vi "1_PrendeLed_Boton.vi"() -> ()   [LabVIEW 2020]
panel:
  out "Boolean array":bool[](array[boolean])
  in  "stop":bool
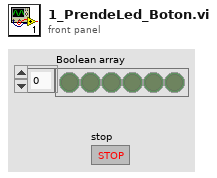
[diagram p1: front panel]
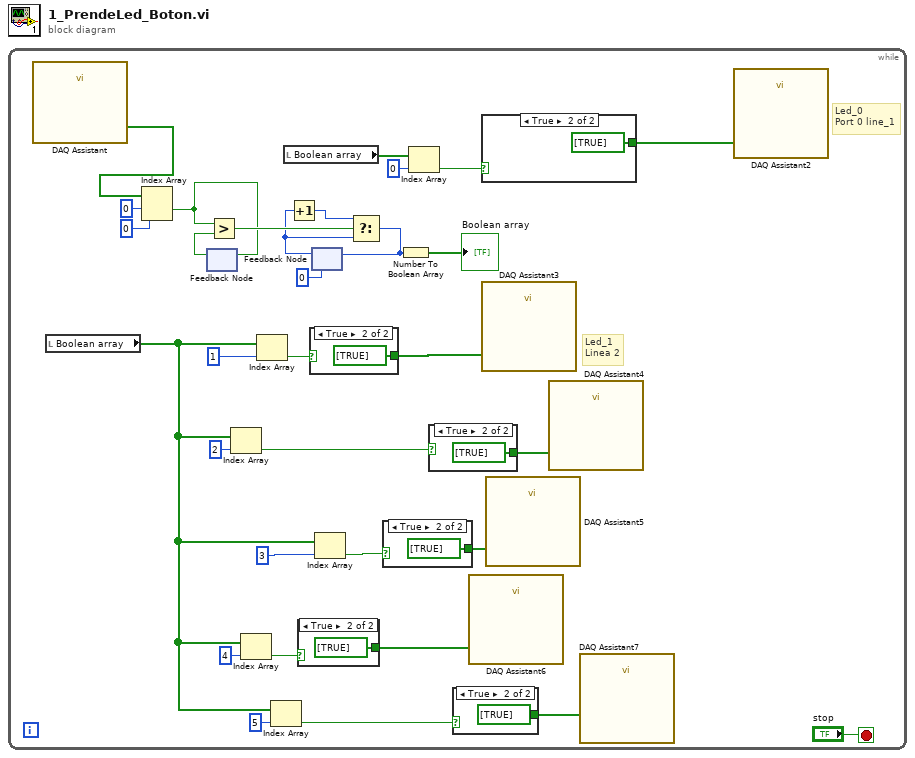
[diagram p0: block diagram]
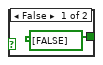
[diagram p2: hidden frame]
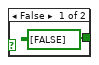
[diagram p3: hidden frame]
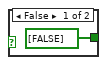
[diagram p4: hidden frame]
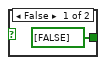
[diagram p5: hidden frame]
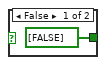
[diagram p6: hidden frame]
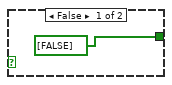
[diagram p7: hidden frame]
diagram:
  n1 = while {
    stop <- "stop" stop-if-true
    # "Led_0\nPort 0 line_1"
    # "Led_1\nLinea 2"
    n2 = call "DAQ Assistant"() -> ("data"=w7:bool[])  [unwired: 17 in, 2 out]
    n3 = local read "Boolean array"() -> (w15:bool[])
    n4 = Index Array(array=w7, index #1=0 ("index"), index #2=0 ("index")) -> (element #1=w9:bool)  [unwired: 1 out]
    n5 = feedback #1() -> (w13:bool)  [unwired: 1 in]
    n6 = feedback-in #1(w9) -> ()
    n7 = Greater?(x=w9, y=w13) -> (0:w14:bool)
    n8 = Index Array(array=w15, index=2) -> (element=w22:bool)
    n9 = Index Array(array=w15, index=4) -> (element=w18:bool)
    n10 = Index Array(array=w15, index=1) -> (element=w24:bool)
    n11 = Index Array(array=w15, index=5) -> (element=w16:bool)
    n12 = local read "Boolean array"() -> (w27:bool[])
    n13 = case shown="True" w18 {
      tunnel: [bool[] [FALSE] ("data") bool[] [TRUE] ("data")] -> w2
      frame False {
      }
      frame True {
      }
    }
    n14 = case shown="True" w24 {
      tunnel: [bool[] [FALSE] ("data") bool[] [TRUE] ("data")] -> w5
      frame False {
      }
      frame True {
      }
    }
    n15 = feedback #2(0) -> (w11:i32)
    n16 = Increment(x=w11) -> (x+1=w10:i32)
    n17 = Index Array(array=w15, index=3) -> (element=w20:bool)
    n18 = Select(t=w10, s=w14, f=w11) -> (s? t:f=w8:i32)
    n19 = feedback-in #2(w8) -> ()
    n20 = case shown="True" w20 {
      tunnel: [bool[] [FALSE] ("data") bool[] [TRUE] ("data")] -> w3
      frame False {
      }
      frame True {
      }
    }
    n21 = Number To Boolean Array(number=w8) -> (Boolean array=→"Boolean array":bool[])
    n22 = Index Array(array=w27, index=0) -> (element=w26:bool)
    n23 = case shown="True" w22 {
      tunnel: [bool[] [FALSE] ("data") bool[] [TRUE] ("data")] -> w4
      frame False {
      }
      frame True {
      }
    }
    n24 = case shown="True" w16 {
      tunnel: [bool[] [FALSE] ("data") bool[] [TRUE] ("data")] -> w1
      frame False {
      }
      frame True {
      }
    }
    n25 = call "DAQ Assistant6"("data"=w2) -> ()  [unwired: 17 in, 2 out]
    n26 = case shown="True" w26 {
      tunnel: [bool[] [FALSE] ("data") bool[] [TRUE] ("data")] -> w6
      frame False {
      }
      frame True {
      }
    }
    n27 = call "DAQ Assistant3"("data"=w5) -> ()  [unwired: 17 in, 2 out]
    n28 = call "DAQ Assistant5"("data"=w3) -> ()  [unwired: 17 in, 2 out]
    n29 = call "DAQ Assistant4"("data"=w4) -> ()  [unwired: 17 in, 2 out]
    n30 = call "DAQ Assistant7"("data"=w1) -> ()  [unwired: 17 in, 2 out]
    n31 = call "DAQ Assistant2"("data"=w6) -> ()  [unwired: 17 in, 2 out]
  }
